vi "QVA_AppendAttribute.vi"(0 "QueueIn":refnum<queue>, 1 "Name":string, 2 "Type":string="unknown", 3 "VariantData":variant, 5 "ErrorIn":errorcluster, 7 "SkipForExistingVariableName":bool, 9 "Timeout":i32=-1) -> (14 "QueueOut":refnum<queue>, 16 "Timeout":bool, 19 "ErrorOut":errorcluster)   [LabVIEW 2016]
doc: "Schreibt eine Variable und die Variant Attributes des Single Element Queues, oder ersetzt eine bereits vorhandene (ausser Option SkipForExistingVariableName = TRUE)\n\nsige / 3.12.13"
uses:
  private/QVA.VariableDataTypeDef.ctl
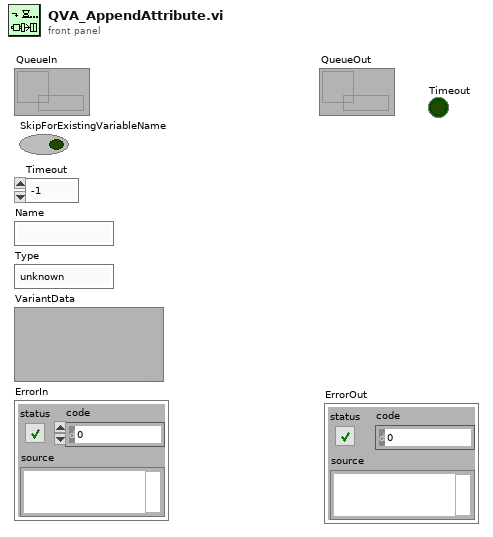
[diagram p1: front panel]
types:
  T1 = typedef "QVA.VariableDataTypeDef.ctl" = cluster{"Type":string, "Data":variant}
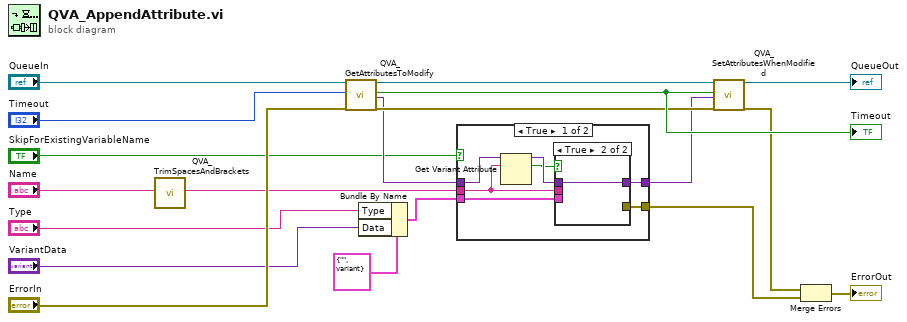
[diagram p0: block diagram]
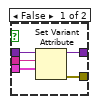
[diagram p2: hidden frame]
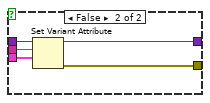
[diagram p3: hidden frame]
diagram:
  n1 = call "QVA_TrimSpacesAndBrackets.vi"("String"="Name") -> ("TrimmedString"=w4:string)  [unwired: 18 in]
  n2 = call "QVA_GetAttributesToModify.vi"("QueueIn"="QueueIn", "Timeout"="Timeout", "ErrorIn"="ErrorIn") -> ("QueueOut"=w19:refnum<queue>, "Timeout"=w15:bool, "VariantData"=w2:variant, "ErrorOut"=w10:errorcluster)  [unwired: 13 in]
  "Timeout" <- w15
  n3 = Bundle By Name(cluster=T1 {"Type"="", "Data"=variant} ("Cluster"), "Type"="Type", "Data"="VariantData") -> (w9:T1)
  n4 = case shown="True" "SkipForExistingVariableName" {
    tunnel: w9 -> [w26 w37]
    tunnel: [w25 w36] -> w6
    tunnel: w2 -> [w23 w35]
    tunnel: w4 -> [w22 w34]
    tunnel: [w24 w33] -> w3
    frame True {
      n5 = Get Variant Attribute(Variant=w23, name=w22) -> (duplicate Variant=w21:variant, found=w20:bool)  [unwired: 2 in, 2 out]
      n6 = case shown="True" w20 {
        tunnel: w26 -> [w31 _]
        tunnel: [w30 _] -> w25
        tunnel: [w29 w32] -> w24
        tunnel: w22 -> [w28 _]
        tunnel: w21 -> [w27 w32]
        frame False {
          n7 = Set Variant Attribute(Variant=w27, name=w28, value=w31) -> (Variant out=w29:variant, error out=w30:errorcluster)  [unwired: 1 in, 1 out]
        }
        frame True {
        }
      }
    }
    frame False {
      n8 = Set Variant Attribute(Variant=w35, name=w34, value=w37) -> (Variant out=w33:variant, error out=w36:errorcluster)  [unwired: 1 in, 1 out]
    }
  }
  n9 = call "QVA_SetAttributesWhenModified.vi"("QueueIn"=w19, "SkipAfterTimeout"=w15, "VariantData"=w3, "ErrorIn"=w10) -> ("QueueOut"=→"QueueOut":refnum<queue>, "ErrorOut"=w13:errorcluster)  [unwired: 14 in]
  n10 = Merge Errors(w13, w6) -> (→"ErrorOut":errorcluster)
